vi "sample6(BulkRW All).vi"() -> ()   [LabVIEW 2011]
panel:
  out "BulkRead Data":T1(array[cluster]) {"Error" format="%04x"}
  out "ACK3":bool
  out "ACK2":bool
  out "ACK1":bool
  in  "UPDATE":bool
  in  "STOP":bool
  in  "TorqueEnable":bool
  in  "OffsetTime":u32=20
  in  "id3":u8=3 max=253
  in  "id2":u8=2 max=253
  in  "id1":u8=1 max=253
  in  "pos3":i32(knob) scale=131594.0..-131594.0
  in  "pos2":i32(knob) scale=131594.0..-131594.0
  in  "pos1":i32(knob) scale=131594.0..-131594.0
  in  "COM":refnum<visa-resource-name> caption="COMポート"
  in  "Baudrate":u32=1000000
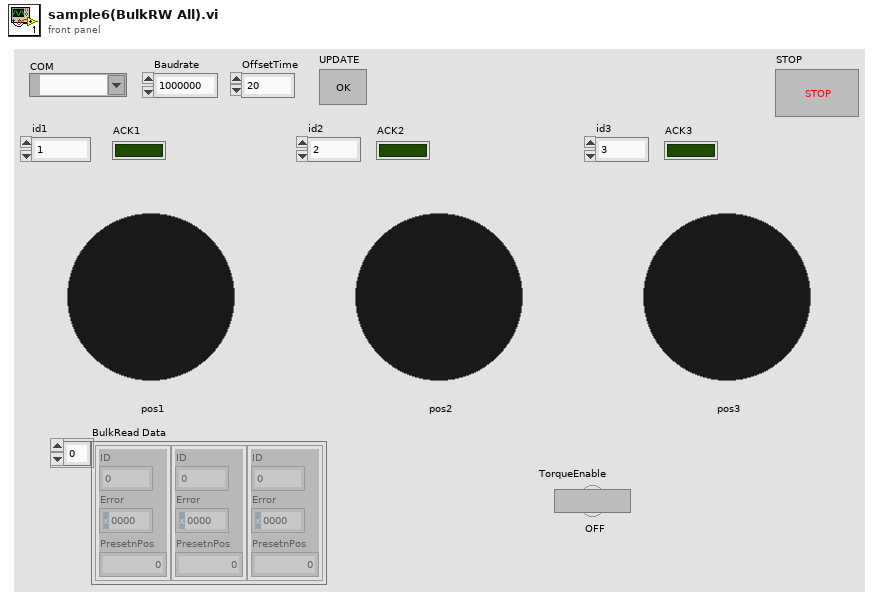
[diagram p1: front panel]
types:
  T1 = cluster{"ID":u8, "Error":u16, "PresetnPos":i32}[]
  T2 = cluster{"ID":u8, "address":u16, "width":u8, "array":u8[]}[]
  T3 = cluster{"ACK":bool, "ID":u8, "MaxPositionLimit":cluster{"address":u16, "width":u8, "limit":cluster{"max":i32, "min":i32}}, "MinPositionLimit":cluster{"address":u16, "width":u8, "limit":cluster{"max":i32, "min":i32}}, "TorqueEnable":cluster{"address":u16, "width":u8, "limit":cluster{"max":i32, "min":i32}}, "GoalPosition":cluster{"address":u16, "width":u8, "limit":cluster{"max":i32, "min":i32}}, "GoalVelocity":cluster{"address":u16, "width":u8, "limit":cluster{"max":i32, "min":i32}}, "PresentPosition":cluster{"address":u16, "width":u8, "limit":cluster{"max":i32, "min":i32}}, "PresentVelocity":cluster{"address":u16, "width":u8, "limit":cluster{"max":i32, "min":i32}}, "HardwareError":cluster{"address":u16, "width":u8, "limit":cluster{"max":i32, "min":i32}}}
  T4 = cluster{"ACK":bool, "ID":u8, "MaxPositionLimit":cluster{"address":u16, "width":u8, "limit":cluster{"max":i32, "min":i32}}, "MinPositionLimit":cluster{"address":u16, "width":u8, "limit":cluster{"max":i32, "min":i32}}, "TorqueEnable":cluster{"address":u16, "width":u8, "limit":cluster{"max":i32, "min":i32}}, "GoalPosition":cluster{"address":u16, "width":u8, "limit":cluster{"max":i32, "min":i32}}, "GoalVelocity":cluster{"address":u16, "width":u8, "limit":cluster{"max":i32, "min":i32}}, "PresentPosition":cluster{"address":u16, "width":u8, "limit":cluster{"max":i32, "min":i32}}, "PresentVelocity":cluster{"address":u16, "width":u8, "limit":cluster{"max":i32, "min":i32}}, "HardwareError":cluster{"address":u16, "width":u8, "limit":cluster{"max":i32, "min":i32}}}[]
  T5 = cluster{"ID":u8, "address":u16, "width":u8, "array":u8[]}
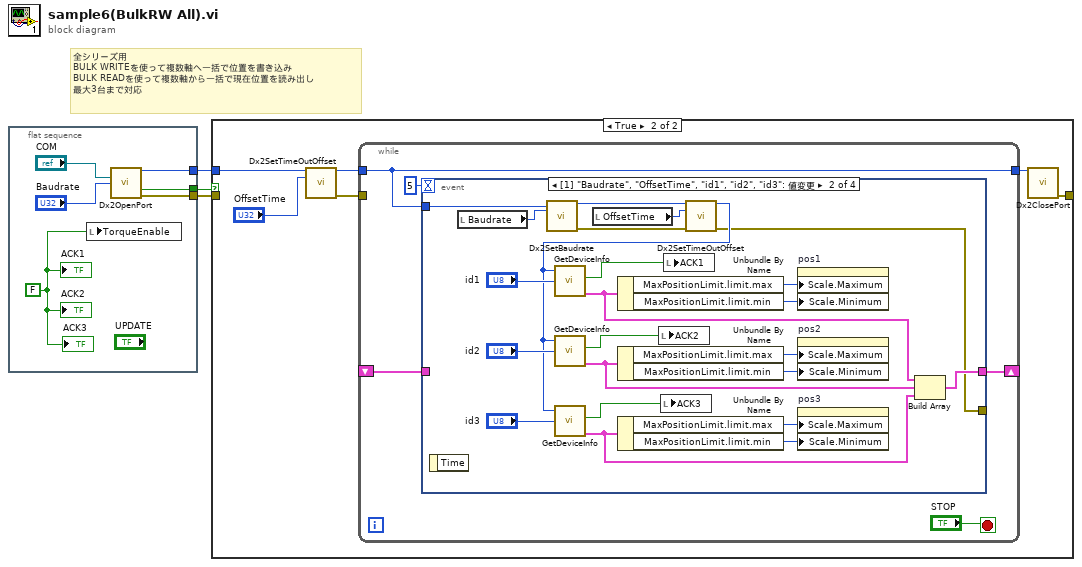
[diagram p0: block diagram]
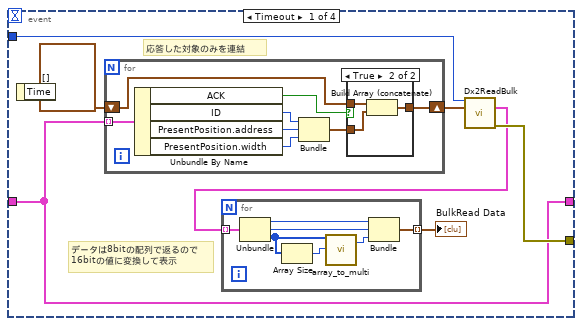
[diagram p3: hidden frame]
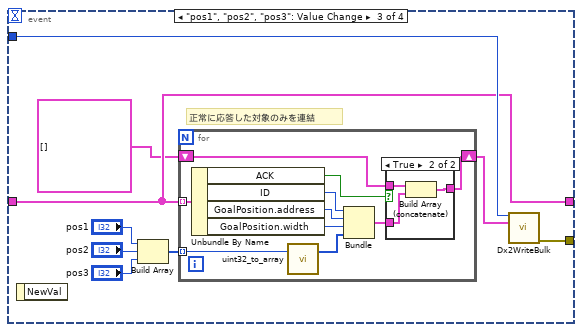
[diagram p5: hidden frame]
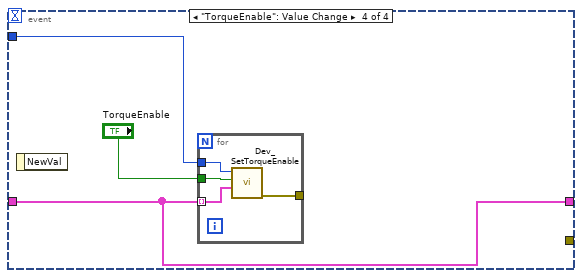
[diagram p7: hidden frame]
diagram:
  # "全シリーズ用\nBULK WRITEを使って複数軸へ一括で位置を書き込み\nBULK READを使って複数軸から一括で現在位置を読み出し\n最大3台まで対応"
  n1 = flat-sequence {
    tunnel: [w7] -> w3
    tunnel: [w6] -> w2
    tunnel: [w5] -> w1
    frame #0 {
      w4 = FALSE
      n2 = local write "TorqueEnable"(w4) -> ()
      n3 = call "Dx2OpenPort.vi"("port"="COM", "baudrate"="Baudrate") -> ("dvid"=w5:u32, "成功"=w7:bool, "エラー出力"=w6:errorcluster)  [unwired: 11 in]
      "ACK1" <- w4
      "ACK2" <- w4
      "ACK3" <- w4
    }
  }
  n4 = case shown="TRUE" w3 {
    tunnel: w1 -> [_ w15]
    tunnel: w2 -> [_ _]
    tunnel: [_ w10] -> _
    frame False {
    }
    frame True {
      n5 = call "Dx2SetTimeOutOffset.vi"("dvid in"=w15, "OffsetTime"="OffsetTime") -> ("dvid out"=w13:u32, "エラー出力"=w12:errorcluster)  [unwired: 12 in]
      n6 = while {
        shift-right: [w20] -> _
        shift-left: _ -> [w19]
        tunnel: w13 -> [w18]
        tunnel: [w18] -> w11
        tunnel: w12 -> [_]
        stop <- "STOP" stop-if-true
        n7 = event shown="[1] \"Baudrate\", \"OffsetTime\", \"id1\", \"id2\", \"id3\": 値変更" {
          selector: _ -> [_ _ _ _]
          dyn-events: _ -> [_ _ _ _]
          timeout: 5 -> [_ _ _ _]
          tunnel: [w25 w55 w72 w93] -> w20
          tunnel: w18 -> [w27 w63 w78 w95]
          tunnel: w19 -> [w25 _ w72 w93]
          tunnel: [w26 w47 w77 _] -> _
          event Timeout {
            # "データは8bitの配列で返るので\n16bitの値に変換して表示"
            # "応答した対象のみを連結"
            n8 = event-data() -> ()  [unwired: 1 in, 1 out]
            n9 = for {
              tunnel: w25 -> [w37] mode=indexing
              shift-right: [w36] -> w23
              shift-left: cluster{"ID":u8, "address":u16, "width":u8}[] [] -> [w35]
              n10 = Unbundle By Name(w37) -> ("ACK"=w39:bool, "ID"=w42:u8, "PresentPosition.address"=w41:u16, "PresentPosition.width"=w40:u8)
              n11 = Bundle("ID"=w42, "address"=w41, "width"=w40) -> (w38:cluster{"ID":u8, "address":u16, "width":u8})  [unwired: 1 in]
              n12 = case shown="TRUE" w39 {
                tunnel: w38 -> [_ w46]
                tunnel: [w43 w45] -> w36
                tunnel: w35 -> [w43 w44]
                frame False {
                }
                frame True {
                  n13 = Build Array (concatenate)(w44, w46) -> (w45:cluster{"ID":u8, "address":u16, "width":u8}[])
                }
              }
            }
            n14 = call "Dx2ReadBulk.vi"("dvid in"=w27, "Param"=w23) -> ("data out"=w21:cluster{"ID":u8, "Error":u16, "Data":u8[]}[], "エラー出力"=w26:errorcluster)  [unwired: 10 in, 2 out]
            n15 = for {
              tunnel: w21 -> [w34] mode=indexing
              tunnel: [w30] -> w22 mode=indexing
              n16 = Unbundle(w34) -> ("ID"=w31:u8, "Error"=w32:u16, "Data"=w29:u8[])
              n17 = Array Size(array=w29) -> (size(s)=w28:i32)
              n18 = call "array_to_multi.vi"("array"=w29, "length"=w28) -> ("uint32"=w33:u32)  [unwired: 17 in]
              n19 = Bundle("ID"=w31, "Error"=w32, "uint32"=w33) -> (w30:cluster{"ID":u8, "Error":u16, "uint32":u32})  [unwired: 1 in]
            }
            "BulkRead Data" <- w22
          }
          event "Baudrate", "OffsetTime", "id1", "id2", "id3": Value Change {
            n20 = event-data() -> ()  [unwired: 1 in, 1 out]
            n21 = local read "Baudrate"() -> (w62:u32)
            n22 = call "Dx2SetBaudrate.vi"("dvid in"=w63, "Baudrate"=w62) -> ("dvid out"=w51:u32, "エラー出力"=w48:errorcluster)  [unwired: 11 in, 1 out]
            n23 = local read "OffsetTime"() -> (w49:u32)
            n24 = call "Dx2SetTimeOutOffset.vi"("dvid in"=w51, "OffsetTime"=w49, "エラー入力"=w48) -> ("dvid out"=w50:u32, "エラー出力"=w47:errorcluster)  [unwired: 11 in]
            n25 = call "GetDeviceInfo.vi"("dvid in"=w50, "Target ID"="id1") -> ("matched"=w58:bool, "ItemInfo"=w54:T3)  [unwired: 1 in, 2 out]
            n26 = call "GetDeviceInfo.vi"("dvid in"=w50, "Target ID"="id2") -> ("matched"=w57:bool, "ItemInfo"=w53:T3)  [unwired: 1 in, 2 out]
            n27 = call "GetDeviceInfo.vi"("dvid in"=w50, "Target ID"="id3") -> ("matched"=w56:bool, "ItemInfo"=w52:T3)  [unwired: 1 in, 2 out]
            n28 = Unbundle By Name(w54) -> ("MaxPositionLimit.limit.max"=w64:i32, "MaxPositionLimit.limit.min"=w65:i32)
            n29 = Unbundle By Name(w53) -> ("MaxPositionLimit.limit.max"=w66:i32, "MaxPositionLimit.limit.min"=w67:i32)
            n30 = Unbundle By Name(w52) -> ("MaxPositionLimit.limit.max"=w68:i32, "MaxPositionLimit.limit.min"=w69:i32)
            n31 = local write "ACK2"(w57) -> ()
            n32 = local write "ACK3"(w56) -> ()
            n33 = local write "ACK1"(w58) -> ()
            n34 = property on="pos1" class="Knob （指定）"("Scale.Maximum"=w64, "Scale.Minimum"=w65) -> ()  [unwired: 2 in, 2 out]
            n35 = property on="pos2" class="Knob （指定）"("Scale.Maximum"=w66, "Scale.Minimum"=w67) -> ()  [unwired: 2 in, 2 out]
            n36 = property on="pos3" class="Knob （指定）"("Scale.Maximum"=w68, "Scale.Minimum"=w69) -> ()  [unwired: 2 in, 2 out]
            n37 = Build Array(w54, w53, w52) -> (w55:T4)
          }
          event "pos1", "pos2", "pos3": Value Change {
            # "正常に応答した対象のみを連結"
            n38 = event-data() -> ()  [unwired: 1 in, 1 out]
            n39 = Build Array("pos1", "pos2", "pos3") -> (w76:i32[])
            n40 = for {
              tunnel: w76 -> [w82] mode=indexing
              tunnel: w72 -> [w81] mode=indexing
              shift-right: [w80] -> w71
              shift-left: T2 [] -> [w79]
              n41 = Unbundle By Name(w81) -> ("ACK"=w84:bool, "ID"=w86:u8, "GoalPosition.address"=w87:u16, "GoalPosition.width"=w88:u8)
              n42 = call "uint32_to_array.vi"("uint32"=w82) -> ("array"=w85:u8[])  [unwired: 2 in]
              n43 = Bundle("ID"=w86, "address"=w87, "width"=w88, "array"=w85) -> (w83:T5)  [unwired: 1 in]
              n44 = case shown="TRUE" w84 {
                tunnel: w83 -> [_ w92]
                tunnel: [w89 w91] -> w80
                tunnel: w79 -> [w89 w90]
                frame False {
                }
                frame True {
                  n45 = Build Array (concatenate)(w90, w92) -> (w91:T2)
                }
              }
            }
            n46 = call "Dx2WriteBulk.vi"("dvid in"=w78, "data in"=w71) -> ("エラー出力"=w77:errorcluster)  [unwired: 11 in, 2 out]
          }
          event "TorqueEnable": Value Change {
            n47 = event-data() -> ()  [unwired: 1 in, 1 out]
            n48 = for {
              tunnel: w95 -> [w99]
              tunnel: "TorqueEnable" -> [w98]
              tunnel: w93 -> [w97] mode=indexing
              tunnel: [w96] -> _
              n49 = call "Dev_SetTorqueEnable.vi"("ItemInfo"=w97, "torque enable"=w98, "dvid in"=w99) -> ("エラー出力"=w96:errorcluster)  [unwired: 2 in, 2 out]
            }
          }
        }
      }
      n50 = call "Dx2ClosePort.vi"("dvid"=w11) -> ("エラー出力"=w10:errorcluster)  [unwired: 13 in, 1 out]
    }
  }
